vi "Remove Datatype Group.vi"(8 "error in (no error)":errorcluster, 10 "name":string, 11 "Channel group in":refnum<class "Channel group.lvclass">) -> (0 "error out":errorcluster, 2 "found":bool, 3 "Channel group out":refnum<class "Channel group.lvclass">)   [LabVIEW 2016, in "FPGA RM Shared API.lvlib" / "Channel group.lvclass"]
uses:
  Channel group.lvclass
  Channel group.lvclass/Channel group.ctl
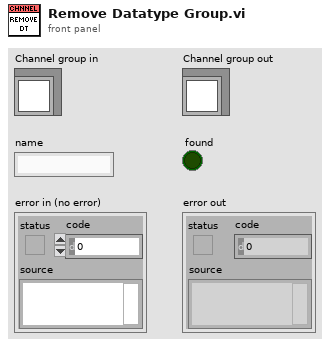
[diagram p1: front panel]
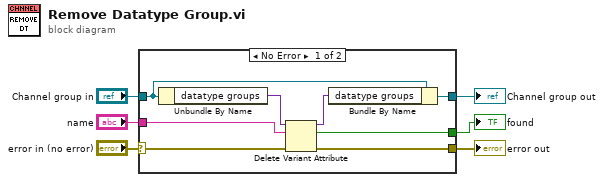
[diagram p0: block diagram]
diagram:
  n1 = case shown="No Error" "error in (no error)" {
    selector: "error in (no error)" -> [w8 w16]
    tunnel: [w7 w16] -> w5
    tunnel: [w13 w15] -> w3
    tunnel: "Channel group in" -> [w14 w15]
    tunnel: "name" -> [w11 _]
    tunnel: [w9 _] -> w1
    frame No Error {
      n2 = Unbundle By Name(w14) -> ("datatype groups"=w12:variant)
      n3 = Delete Variant Attribute(4:w8, 6:w11, 7:w12) -> (0:w7:errorcluster, 2:w9:bool, 3:w10:variant)
      n4 = Bundle By Name(cluster=w14, "datatype groups"=w10) -> (w13:refnum<class "Channel group.lvclass">)
    }
    frame Error {
    }
  }
  "error out" <- w5
  "Channel group out" <- w3
  "found" <- w1
